vi "ini_load_variables.vi"(8 "error in":errorcluster, 11 "objects":refnum<vi>[](array[refnum])) -> (0 "error out":errorcluster)   [LabVIEW 2013]
doc: "Saves referenced objects to INI file. Use this to store last setup of the programm."
uses:
  <vilib>/Utility/config.llb/NI_LVConfig.lvlib
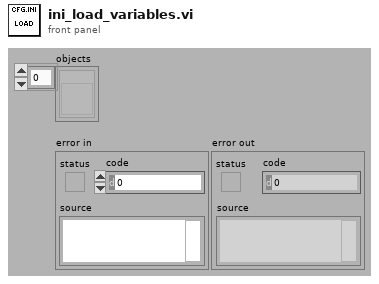
[diagram p1: front panel]
types:
  T1 = typedef "ini_parse_row.ctl" = cluster{"ini section":string, "ini key":string, "ini default":string, "control ref":refnum<vi>, "uid":i32, "vi ref":refnum<vi>}
  T2 = typedef "NI_LVConfig.lvlib/Config Data RefNum.ctl" = refnum<k1>
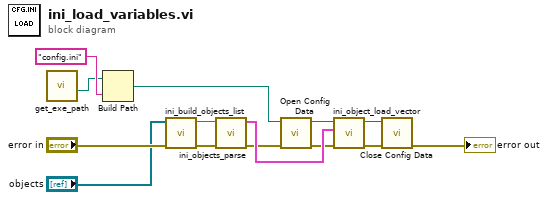
[diagram p0: block diagram]
diagram:
  n1 = call "get_exe_path.vi"() -> ("directory path"=w7:path)  [unwired: 3 out]
  n2 = Build Path(base path=w7, name or relative path="config.ini") -> (appended path=w13:path)
  n3 = call "ini_build_objects_list.vi"("error in"="error in", "objects"="objects") -> ("error out"=w3:errorcluster, "objects list"=w6:string)  [unwired: 8 in]
  n4 = call "ini_objects_parse.vi"("error in"=w3, "items command"=w6) -> ("error out"=w2:errorcluster, "ini items"=w8:T1[])  [unwired: 8 in]
  n5 = call <vilib>:"Open Config Data.vi"("error in (no error)"=w2, "configuration file path"=w13) -> ("error out"=w1:errorcluster, "refnum"=w12:T2)  [unwired: 7 in, 1 out]
  n6 = call "ini_object_load_vector.vi"("error in"=w1, "objects to save"=w8, "refnum in"=w12) -> ("error out"=w11:errorcluster, "refnum out"=w10:T2)  [unwired: 7 in]
  n7 = call <vilib>:"Close Config Data.vi"("error in (no error)"=w11, "refnum"=w10) -> ("error out"=→"error out":errorcluster)  [unwired: 8 in, 1 out]
